vi "Idle.vi"(8 "error in (no error)":errorcluster, 11 "Idle in":refnum<class "Idle.lvclass">) -> (0 "error out":errorcluster, 3 "State out":refnum<class "State Actor.lvclass">)   [LabVIEW 2025, in "User_Console-ATM.lvlib" / "Idle.lvclass"]
uses:
  Idle.lvclass
  <vilib>/ni/Actors/State Actor/State Actor/State Actor.lvclass
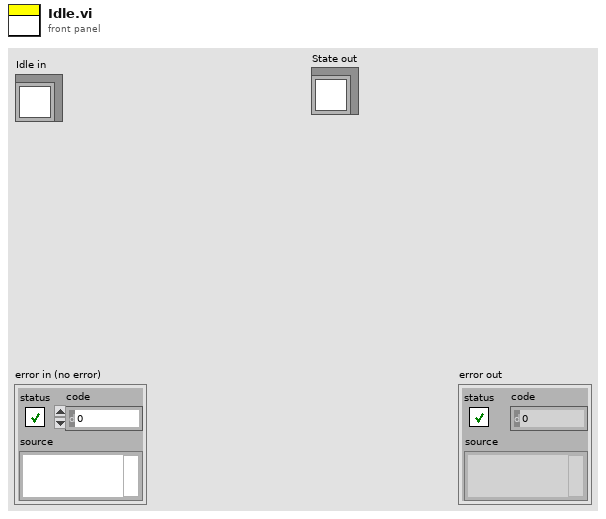
[diagram p1: front panel]
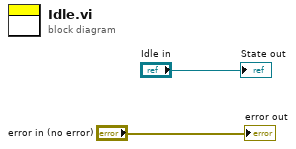
[diagram p0: block diagram]
diagram:
  "error out" <- "error in (no error)"
  "State out" <- "Idle in"
